vi "CSM_0@10.vi"(0 "Qa":dbl, 5 "Pu":dbl, 7 "T":dbl, 9 "Cc":dbl, 11 "q":dbl, 12 "err in":errorcluster) -> (4 "Cpos":dbl, 6 "Cadm":dbl, 8 "CSM":dbl, 14 "err out":errorcluster)   [LabVIEW 2010, in "lv_07.lvlib"]
doc: "Ce VI calcule le coûts de stockage maintenance (CSM) composé du Coût administratif de gestion des commandes (Cadm) et du coût de Possesion (Cpos)."
uses:
  lv_07.lvlib
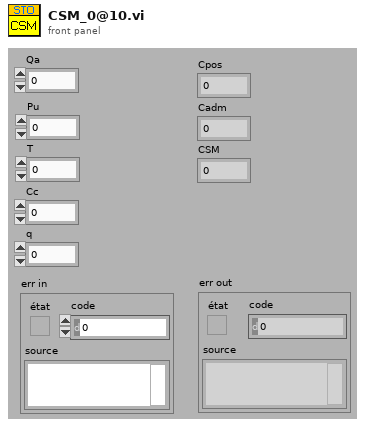
[diagram p1: front panel]
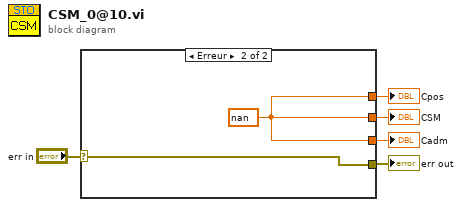
[diagram p0: block diagram]
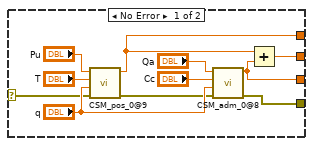
[diagram p2: hidden frame]
diagram:
  n1 = case shown="Erreur" "err in" {
    selector: "err in" -> [w6 w18]
    tunnel: [w12 w17] -> w5
    tunnel: [w11 w17] -> w4
    tunnel: [w10 w17] -> w3
    tunnel: [w8 w18] -> w2
    frame No Error {
      n2 = call "CSM_pos_0@9.vi"("error in (no error)"=w6, "q"="q", "T"="T", "Pu"="Pu") -> ("error out"=w7:errorcluster, "Cpos"=w10:dbl)  [unwired: 2 in]
      n3 = call "CSM_adm_0@8.vi"("err in"=w7, "q"="q", "Cc"="Cc", "Qa"="Qa") -> ("err out"=w8:errorcluster, "Cadm"=w11:dbl)  [unwired: 2 in]
      n4 = Add(x=w10, y=w11) -> (x+y=w12:dbl)
    }
    frame Error {
      w17 = nan
    }
  }
  "CSM" <- w5
  "Cpos" <- w3
  "err out" <- w2
  "Cadm" <- w4
